vi "Chassis Temp.vi"(11 "Desired Temperature Units":i16(ring) items=["Celsius", "Fahrenheit", "Kelvin", "Rankine"]) -> (3 "Chassis Temperature":sgl)   [LabVIEW 2016]
uses:
  <vilib>/rvi/Emulation/niFpgaGetClockAttributes.vi
  <vilib>/rvi/Emulation/niFpgaSctlEmulationGetInTimedLoop.vi
  <vilib>/rvi/Emulation/niFpgaEmulationReportErrorSimple.vi
  <vilib>/rvi/eio/common/nirviEmuTemplateMethod_errors.vi
  <vilib>/rvi/Emulation/niFpgaCriticalErrorInLSC.vi
  <vilib>/eio/EIONode/EIONode.xnode
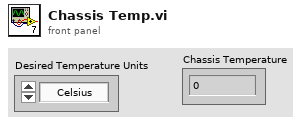
[diagram p1: front panel]
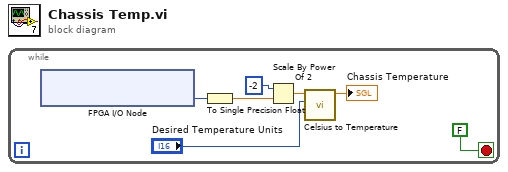
[diagram p0: block diagram]
diagram:
  n1 = while {
    stop <- FALSE stop-if-true
    n2 = xnode "FPGA I/O Node"() -> ("Chassis Temperature"=w2:i16)  [unwired: 1 in, 1 out]
    n3 = To Single Precision Float(number=w2) -> (single precision float=w5:sgl)
    n4 = Scale By Power Of 2(n=i16 -2, x=w5) -> (x*2^n=w3:sgl)
    n5 = call "Celsius to Temperature.vi"("Desired Temperature Units"="Desired Temperature Units", "Input Temperature (*C)"=w3) -> ("Temperature"=→"Chassis Temperature":sgl)  [unwired: 9 in]
  }
